vi "FRCts20_WebMethods_Redirect_Division.vi"(7 "response code (200)":i32(ring)=200 items=["100"=100, "101"=101, "200"=200, "201"=201, "202"=202, "203"=203, "204"=204, "205"=205, "206"=206, "300"=300, "301"=301, "302"=302, "303"=303, "304"=304, "305"=305, "306"=306, "307"=307, "400"=400, "401"=401, "402"=402, "403"=403, "404"=404, "405"=405, "406"=406, "407"=407, "408"=408, "409"=409, "410"=410, "411"=411, "412"=412, "413"=413, "414"=414, "415"=415, "416"=416, "417"=417, "500"=500, "501"=501, "502"=502, "503"=503, "504"=504, "505"=505], 8 "error in (no error)":errorcluster, 10 "Division":T1, 11 "httpRequestID":u32) -> (0 "error out":errorcluster, 3 "httpRequestID out":u32)   [LabVIEW 2013, in "FRCts20_WebMethods.lvlib"]
uses:
  FRCts20_WebMethods.lvlib
  Backend/source/VI Source/FRCts20_Backend_API/FRCts20_Backend_API_Division.ctl
  Backend/source/VI Source/FRCts20_Backend_API/FRCts20_Backend_API_SW.ctl
  Backend/source/VI Source/FRCts20_Backend_API/FRCts20_Backend_API_Status.ctl
  <vilib>/wsapi/NI_WebServices.lvlib
  Backend/source/VI Source/FRCts20_Backend_API/FRCts20_Backend_API.lvlib
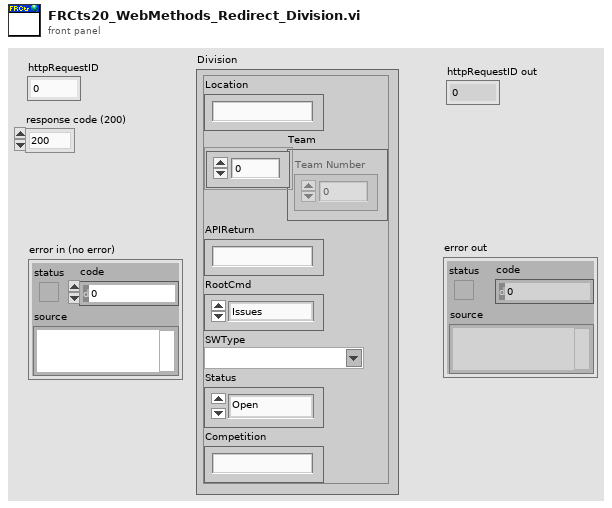
[diagram p1: front panel]
types:
  T1 = typedef "FRCts20_Backend_API.lvlib/FRCts20_Backend_API_Division.ctl" = cluster{"Location":string, "Team":u32[], "APIReturn":string, "RootCmd":enum16{"Issues", "Software", "All"}, "SWType":T2, "Status":T3, "Competition":string}
  T2 = typedef "FRCts20_Backend_API.lvlib/FRCts20_Backend_API_SW.ctl" = string
  T3 = typedef "FRCts20_Backend_API.lvlib/FRCts20_Backend_API_Status.ctl" = enum16{"Open", "In Work", "Closed"}
  T4 = typedef "FRCts20_WebMethods.lvlib/FRCts20_WebMethods_ctl_returntype.ctl" = string
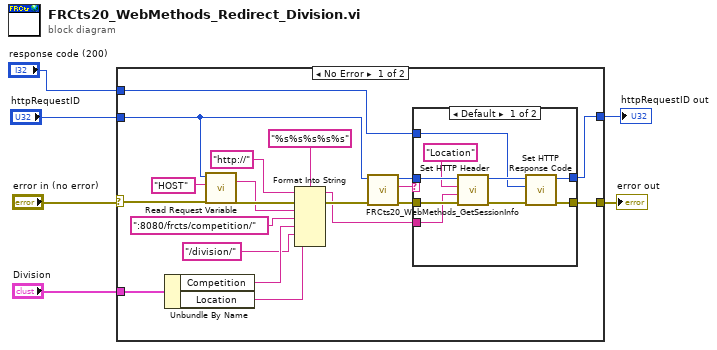
[diagram p0: block diagram]
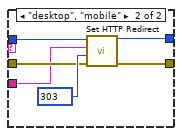
[diagram p2: hidden frame]
diagram:
  n1 = case shown="No Error" "error in (no error)" {
    selector: "error in (no error)" -> [w15 w43]
    tunnel: [w14 w43] -> w6
    tunnel: "httpRequestID" -> [w7 w42]
    tunnel: [w13 w42] -> w4
    tunnel: "Division" -> [w26 _]
    tunnel: "response code (200)" -> [w9 _]
    frame No Error {
      n2 = Unbundle By Name(w26) -> ("Competition"=w20:string, "Location"=w10:string)
      n3 = call <vilib>:"Read Request Variable.vi"("error in (no error)"=w15, "variable name"="HOST", "httpRequestID"=w7) -> ("error out"=w24:errorcluster, "value"=w21:string)  [unwired: 6 in, 1 out]
      n4 = Format Into String(format string="%s%s%s%s%s", initial string="http://", error in=w24, w21, ":8080/frcts/competition/", w20, "/division/", w10) -> (resulting string=w12:string, error out=w16:errorcluster)
      n5 = call "FRCts20_WebMethods_GetSessionInfo.vi"("error in"=w16, "httpRequestID"=w7) -> ("error out"=w18:errorcluster, "Return Type"=w19:T4, "httpRequestID out"=w17:u32)  [unwired: 7 in]
      n6 = case shown="Default" w19 {
        tunnel: [w31 w41] -> w14
        tunnel: [w28 w40] -> w13
        tunnel: w18 -> [w35 w38]
        tunnel: w17 -> [w34 w37]
        tunnel: w12 -> [w32 w36]
        tunnel: w9 -> [w27 _]
        frame Default {
          n7 = call <vilib>:"Set HTTP Header.vi"("error in (no error)"=w35, "header value"=w32, "header"="Location", "httpRequestID"=w34) -> ("error out"=w30:errorcluster, "httpRequestID out"=w29:u32)  [unwired: 6 in]
          n8 = call <vilib>:"Set HTTP Response Code.vi"("error in (no error)"=w30, "response code (200)"=w27, "httpRequestID"=w29) -> ("error out"=w31:errorcluster, "httpRequestID out"=w28:u32)  [unwired: 7 in]
        }
        frame "desktop", "mobile" {
          w39 = 303 items=["100"=100, "101"=101, "200"=200, "201"=201, "202"=202, "203"=203, "204"=204, "205"=205, "206"=206, "300"=300, "301"=301, "302"=302, "303"=303, "304"=304, "305"=305, "306"=306, "307"=307, "400"=400, "401"=401, "402"=402, "403"=403, "404"=404, "405"=405, "406"=406, "407"=407, "408"=408, "409"=409, "410"=410, "411"=411, "412"=412, "413"=413, "414"=414, "415"=415, "416"=416, "417"=417, "500"=500, "501"=501, "502"=502, "503"=503, "504"=504, "505"=505] ("response code (307)")
          n9 = call <vilib>:"Set HTTP Redirect.vi"("error in (no error)"=w38, "response code (307)"=w39, "redirect URL"=w36, "httpRequestID"=w37) -> ("error out"=w41:errorcluster, "httpRequestID out"=w40:u32)  [unwired: 6 in]
        }
      }
    }
    frame Error {
    }
  }
  "error out" <- w6
  "httpRequestID out" <- w4
